vi "SynapseAPI-Set Block.vi"(0 "URL":string="http://localhost:24414", 7 "block":string, 11 "error in (no error)":errorcluster) -> (15 "error out":errorcluster)   [LabVIEW 2020]
uses:
  <vilib>/httpClient/PUTBuffer.vi
  <vilib>/httpClient/LabVIEWHTTPClient.lvlib
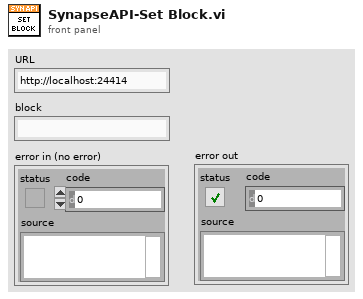
[diagram p1: front panel]
types:
  T1 = typedef "LabVIEWHTTPClient.lvlib/ClientHandle.ctl" = refnum<k1>
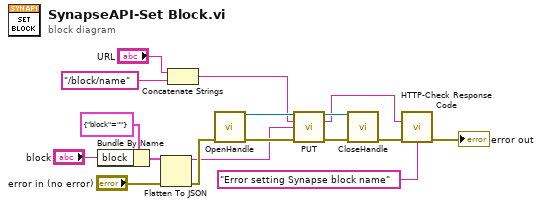
[diagram p0: block diagram]
diagram:
  n1 = Bundle By Name(cluster=cluster{"block":string} {"block"=""} ("Cluster"), "block"="block") -> (w16:cluster{"block":string})
  n2 = Flatten To JSON(anything=w16, error in (no error)="error in (no error)") -> (JSON string=w7:string, 11:w8:errorcluster)  [unwired: 1 in]
  n3 = Concatenate Strings("URL", "/block/name") -> (w9:string)
  n4 = call <vilib>:"OpenHandle.vi"("error in (no error)"=w8) -> ("client handle out"=w12:T1, "error out"=w11:errorcluster)  [unwired: 13 in]
  n5 = call-poly <vilib>:"PUT.vi"("client handle"=w12, "url"=w9, "buffer"=w7, "error in (no error)"=w11) -> ("client handle out"=w14:T1, "headers"=w2:string, "error out"=w15:errorcluster)  [unwired: 8 in, 1 out]
  n6 = call <vilib>:"CloseHandle.vi"("client handle"=w14, "error in (no error)"=w15) -> ("error out"=w4:errorcluster)  [unwired: 13 in]
  n7 = call "HTTP-Check Response Code.vi"("headers"=w2, "error in"=w4, "message"="Error setting Synapse block name") -> ("error out"=→"error out":errorcluster)  [unwired: 12 in]
